vi "Get Temperature.vi"(6 "Channel":i32, 8 "error in (no error)":errorcluster, 11 "instrument.PPMS in":refnum<class "instrument.PPMS3.lvclass">) -> (0 "error out":errorcluster, 1 "Status":variant, 2 "Temperature (K)":dbl, 3 "instrument.PPMS out":refnum<class "instrument.PPMS3.lvclass">, 4 "Finished?":bool)   [LabVIEW 2019, in "instrument.PPMS3.lvclass"]
uses:
  instrument.PPMS3.lvclass
  Typedefs/PPMS3.Commands-enum.ctl
  instrument.PPMS/Typedefs/PPMS.Temperature Status--cluster.ctl
  08798166-d278-40c0-a28b-98a00722a1ce.vi
  08798166-d278-40c0-a28b-98a00722a1ce.vi/b943849a-9cbb-49cf-883d-5cc9bb53a310.vi
  <userlib>/LevyLab/Levylab Instruments/SMOs/RemoteControl/API/Remote Client.vi
  instrument.PPMS/instrument.PPMS.lvclass
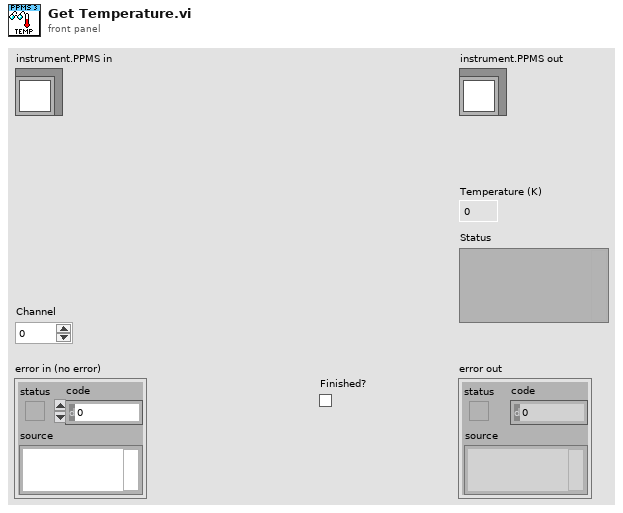
[diagram p1: front panel]
types:
  T1 = typedef "instrument.PPMS.lvclass/PPMS.Temperature Status--cluster.ctl" = cluster{"Temperature (K)":dbl, "Temperature Status":string}
  T2 = typedef "instrument.PPMS3.lvclass/PPMS3.Commands-enum.ctl" = enum16{"Get Magnet Field", "Get Helium Level", "Get Temperature", "Set Magnet Field", "Set Temperature", "getAll"}
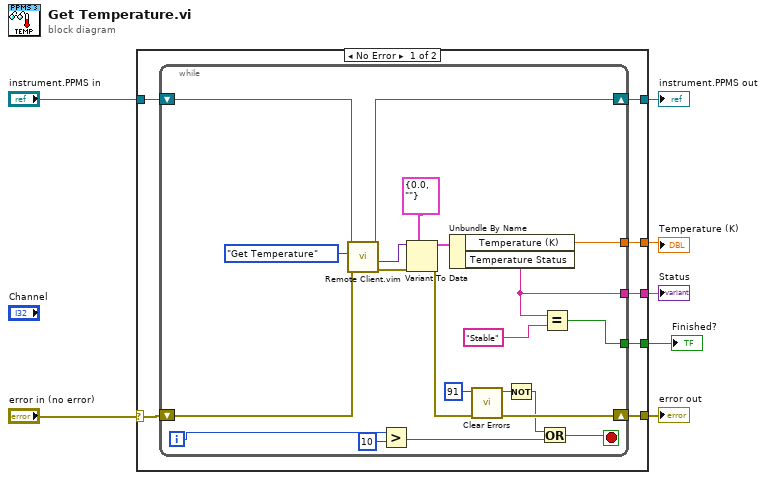
[diagram p0: block diagram]
diagram:
  n1 = case shown="No Error" "error in (no error)" {
    selector: "error in (no error)" -> [w10 w37]
    tunnel: [w14 _] -> w7
    tunnel: [w9 w37] -> w6
    tunnel: [w13 w36] -> w5
    tunnel: "instrument.PPMS in" -> [w12 w36]
    tunnel: [w11 _] -> w3
    tunnel: [w8 _] -> w1
    frame No Error {
      n2 = while {
        tunnel: [w35] -> w14
        tunnel: [w18] -> w11
        shift-right: [w33] -> w13
        shift-left: w12 -> [w32]
        shift-right: [w27] -> w9
        shift-left: w10 -> [w28]
        tunnel: [w16] -> w8
        i -> [w22]
        stop <- w21 stop-if-true
        n3 = call "Remote Client.vim"("error in (no error)"=w28, "Command"=PPMS3.Commands-enum."Get Temperature", "Instrument in"=w32) -> ("error out"=w30:errorcluster, "Data out"=w29:variant, "Instrument out"=w33:refnum<class "instrument.PPMS3.lvclass">)  [unwired: 5 in, 1 out]
        n4 = Greater?(x=w22, y=10) -> (0:w23:bool)
        n5 = Variant To Data(error in=w30, type=T1 {"Temperature (K)"=0.0, "Temperature Status"=""} ("Temperature Status"), Variant=w29) -> (data=w31:T1, error out=w34:errorcluster)
        n6 = Unbundle By Name(w31) -> ("Temperature (K)"=w35:dbl, "Temperature Status"=w18:string)
        n7 = call <vilib>:"Clear Errors.vi"("error in (no error)"=w34, "specific error code to clear (0: all)"=91) -> ("error out"=w27:errorcluster, "specific error cleared?"=w20:bool)  [unwired: 4 in]
        n8 = Not(x=w20) -> (.not. x?=w19:bool)
        n9 = Or(x=w19, y=w23) -> (x .or. y?=w21:bool)
        n10 = Equal?(x=w18, y="Stable" ("Temperature Status")) -> (x = y?=w16:bool)
      }
    }
    frame Error {
    }
  }
  "error out" <- w6
  "instrument.PPMS out" <- w5
  "Temperature (K)" <- w7
  "Status" <- w3
  "Finished?" <- w1
